vi "Add ColumnHead Items by Text Array and ImageIndex Array.vi"(8 "error in (no error)":errorcluster caption="错误输入（无错误）", 9 "ImageIndex":i32[](array[numeric]), 10 "Text":string[](array[string]), 11 "ListViewClass 输入":refnum<class "ListViewClass.lvclass"> caption="DNL_LabVIEW Object in") -> (0 "error out":errorcluster caption="错误输出", 3 "ListViewClass 输出":refnum<class "ListViewClass.lvclass"> caption="DNL_LabVIEW Object out")   [LabVIEW 2012, in "ListViewClass.lvclass"]
uses:
  ListViewClass.lvclass
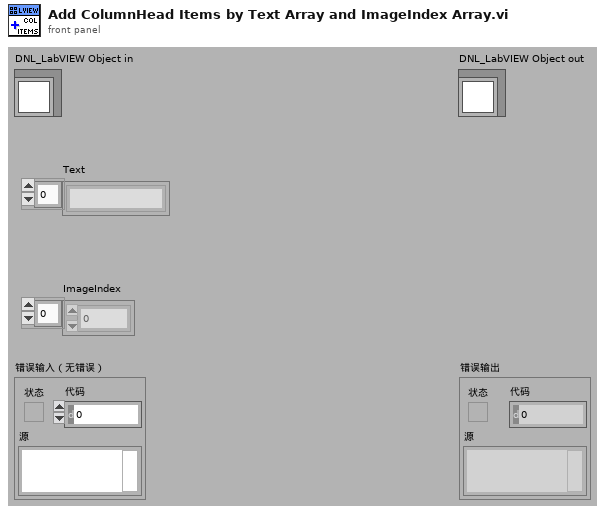
[diagram p1: front panel]
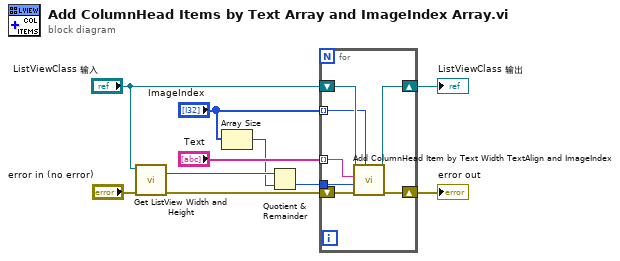
[diagram p0: block diagram]
diagram:
  n1 = call "Get ListView Width and Height.vi"("error in (no error)"="error in (no error)", "ListViewClass 输入"="ListViewClass 输入") -> ("error out"=w1:errorcluster, "Width"=w5:i32)  [unwired: 6 in, 2 out]
  n2 = Array Size(array="ImageIndex") -> (size(s)=w4:i32)
  n3 = Quotient & Remainder(x=w5, y=w4) -> (floor(x/y)=w3:i32)  [unwired: 1 out]
  n4 = for {
    shift-right: [w12] -> w9
    shift-left: "ListViewClass 输入" -> [w17]
    shift-right: [w14] -> w10
    shift-left: w1 -> [w15]
    tunnel: "Text" -> [w16] mode=indexing
    tunnel: "ImageIndex" -> [w13] mode=indexing
    tunnel: w3 -> [w11]
    n5 = call "Add ColumnHead Item by Text Width TextAlign and ImageIndex.vi"("textAlign"=w13, "error in (no error)"=w15, "width"=w11, "text"=w16, "ListViewClass 输入"=w17) -> ("error out"=w14:errorcluster, "ListViewClass 输出"=w12:refnum<class "ListViewClass.lvclass">)  [unwired: 5 in]
  }
  "error out" <- w10
  "ListViewClass 输出" <- w9
